vi "FPGA RS232 Write Read Example.vi"() -> ()   [LabVIEW 2012]
doc: "This VI transfers data to and from the FPGA VI to send and receive bytes from a serial port."
panel:
  out "error out":errorcluster
  out "String read":string
  # "This example is configured to run on a Single-board RIO 9631.  If you have a different RIO device, you\nmust add the appropriate RIO targets to your LabVIEW Project and move the VIs in this project to the new\ntarget.  You must also configure the IP address of the RIO target to match your network configuration.\nFor more information, select Help>>Search the LabVIEW Help and browse to the\nRobotics Module>>Reusing Robotics Examples topics on the Contents tab of the LabVIEW Help.\n\nYou will also need to rename any I/O under the new FPGA target to match the name configured for the\nexample target."
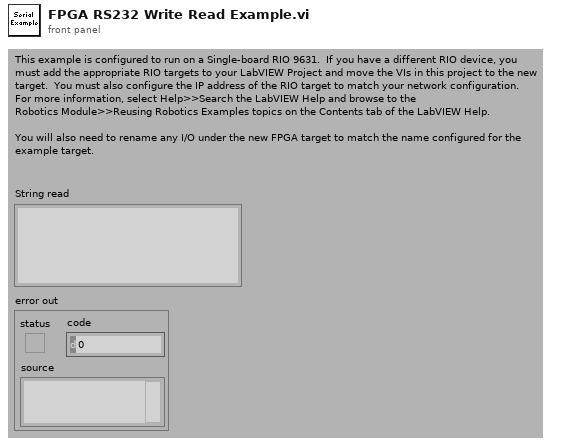
[diagram p1: front panel]
types:
  T1 = typedef "FPGA Main VI Reference Typedef.ctl" = refnum<k20>
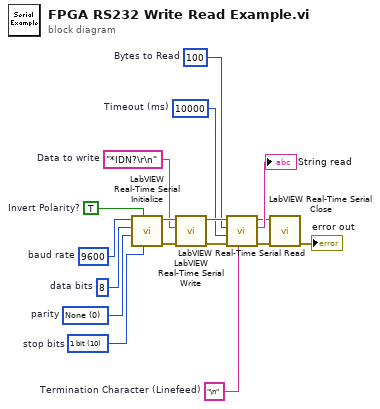
[diagram p0: block diagram]
diagram:
  w1 = u16 10 items=["1 bit"=10, "1.5 bits"=15, "2 bits"=20]  # stop bits
  w2 = u16 0 items=["None", "Odd", "Even", "Mark", "Space"]  # parity
  w3 = u16 8  # data bits
  w4 = TRUE  # Invert Polarity?
  w5 = "\n"  # Termination Character (Linefeed)
  w6 = 10000  # Timeout (ms)
  w11 = u32 100  # Bytes to Read
  w15 = "*IDN?\r\n"  # Data to write
  w17 = u32 9600  # baud rate
  n1 = call "LabVIEW Real-Time Serial Initialize.vi"("stop bits (10: 1 bit)"=w1, "Invert Polarity?"=w4, "parity (0:none)"=w2, "data bits (8)"=w3, "baud rate (9600)"=w17) -> ("error out"=w14:errorcluster, "FPGA VI Reference Out"=w16:T1)  [unwired: 5 in]
  n2 = call "LabVIEW Real-Time Serial Write.vi"("error in (no error)"=w14, "String"=w15, "FPGA Main VI Reference"=w16) -> ("error out"=w13:errorcluster, "FPGA Main VI Reference Out"=w12:T1)  [unwired: 7 in]
  n3 = call "LabVIEW Real-Time Serial Read.vi"("Termination Character (Linefeed)"=w5, "error in (no error)"=w13, "Timeout (ms) (-1: no timeout)"=w6, "Bytes to Read"=w11, "FPGA Main Ref"=w12) -> ("error out"=w8:errorcluster, "String"=→"String read":string, "FPGA Main Ref Out"=w9:T1)  [unwired: 4 in]
  n4 = call "LabVIEW Real-Time Serial Close.vi"("error out"=w8, "FPGA Main Ref"=w9) -> ("error out"=→"error out":errorcluster)  [unwired: 9 in]
